vi "6 - Get transition sequence data from XY data.vi"() -> ()   [LabVIEW 2013]
uses:
  <vilib>/Utility/file.llb/Read From Spreadsheet File (DBL).vi
panel:
  out "Array":string[][](array[string])
  in  "video number":i32
  in  "startend data":path
  in  "player xy and frame data":path
  in  "player transition data":path
  in  "Number of transitions":i32=5
  out "subpatterns out":string[](array[string])
  out "Sub patterns 2":string[](array[string])
  out "Sub patterns":string[](array[string])
  out "top":string[][](array[string])
  out "bottom":string[][](array[string])
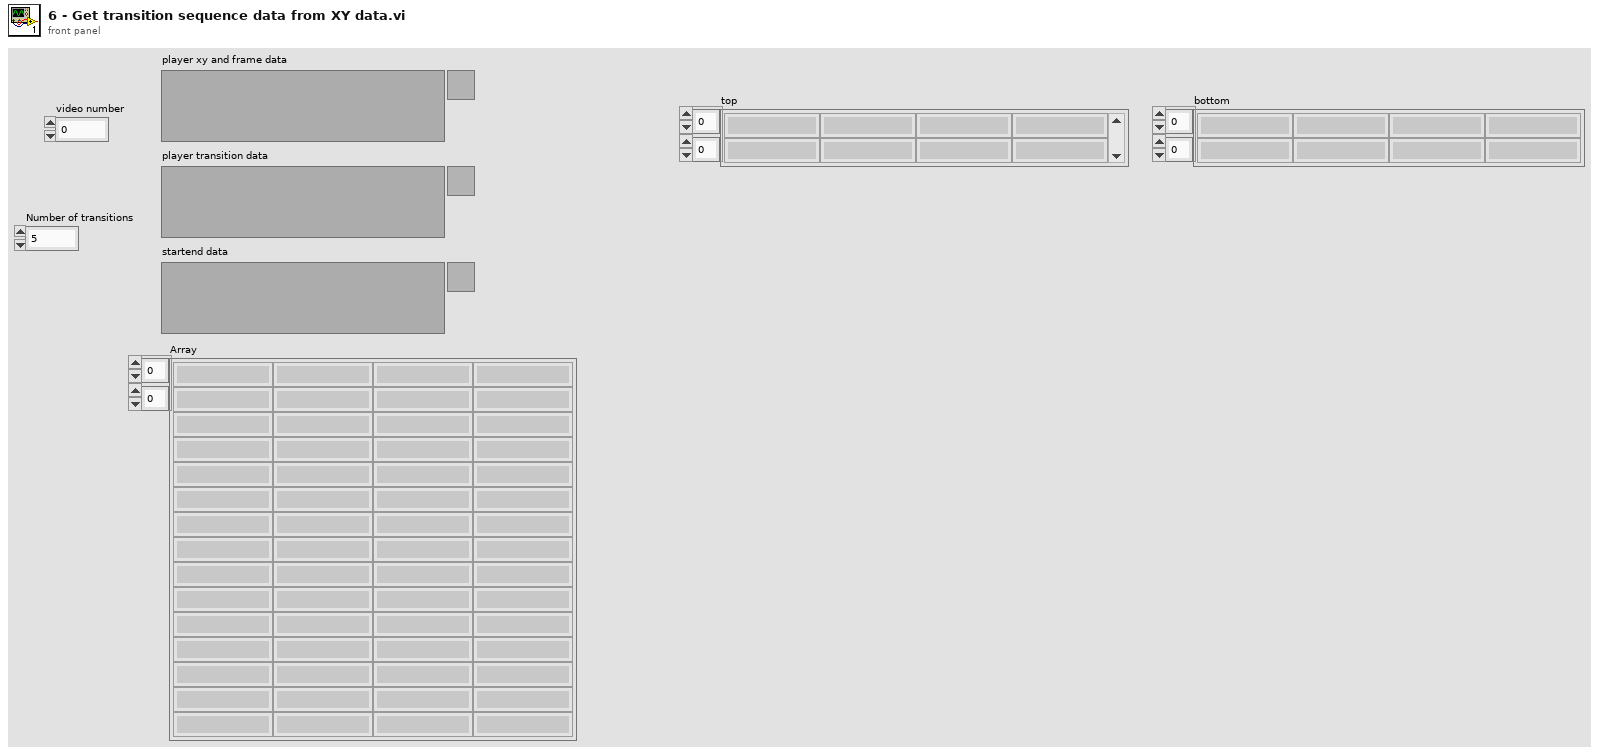
[diagram p1: front panel]
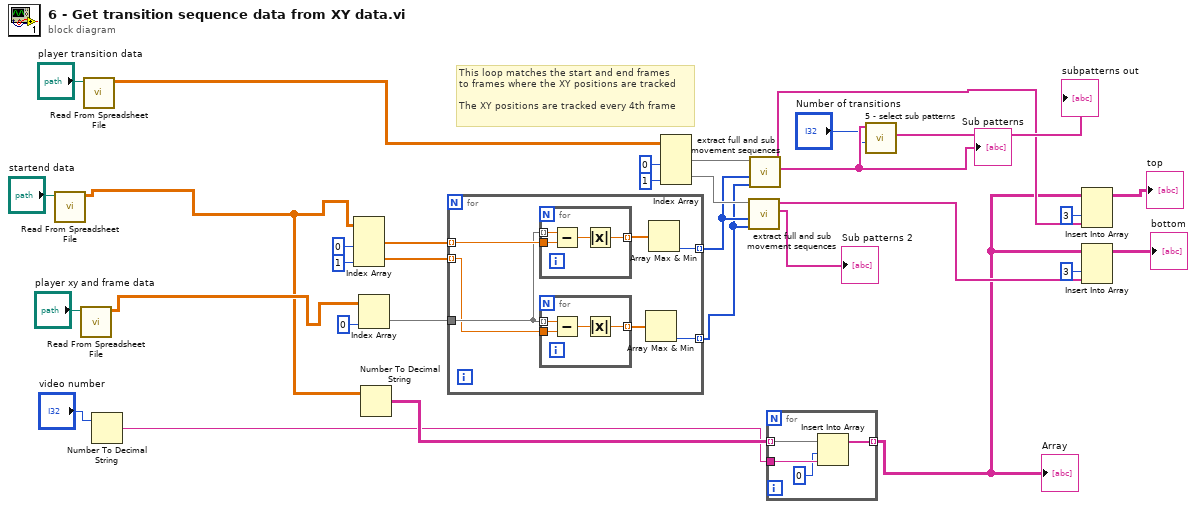
[diagram p0: block diagram]
diagram:
  # "This loop matches the start and end frames \nto frames where the XY positions are tracked\n\nThe XY positions are tracked every 4th frame"
  n1 = call-poly <vilib>:"Read From Spreadsheet File.vi"("file path (dialog if empty)"="startend data") -> ("all rows"=w11:dbl[][])  [unwired: 6 in, 4 out]
  n2 = call-poly <vilib>:"Read From Spreadsheet File.vi"("file path (dialog if empty)"="player xy and frame data") -> ("all rows"=w13:dbl[][])  [unwired: 6 in, 4 out]
  n3 = call-poly <vilib>:"Read From Spreadsheet File.vi"("file path (dialog if empty)"="player transition data") -> ("all rows"=w15:dbl[][])  [unwired: 6 in, 4 out]
  n4 = Number To Decimal String(number="video number") -> (decimal integer string=w8:string)  [unwired: 1 in]
  n5 = Index Array(array=w11, index (col) #1=0 ("disabled index (col)"), index (col) #2=1 ("index (col)")) -> (element #1=w30:dbl[], element #2=w29:dbl[])  [unwired: 2 in]
  n6 = Index Array(array=w13, index (col)=0 ("disabled index (col)")) -> (element=w27:dbl[])  [unwired: 1 in]
  n7 = Number To Decimal String(number=w11) -> (decimal integer string=w9:string[][])  [unwired: 1 in]
  n8 = for {
    tunnel: w30 -> [w39] mode=indexing
    tunnel: w29 -> [w34] mode=indexing
    tunnel: w27 -> [w35]
    tunnel: [w37] -> w22 mode=indexing
    tunnel: [w36] -> w21 mode=indexing
    n9 = for {
      tunnel: w39 -> [w46]
      tunnel: w35 -> [w47] mode=indexing
      tunnel: [w44] -> w38 mode=indexing
      n10 = Subtract(x=w47, y=w46) -> (x-y=w45:dbl)
      n11 = Absolute Value(x=w45) -> (abs(x)=w44:dbl)
    }
    n12 = for {
      tunnel: w34 -> [w42]
      tunnel: w35 -> [w43] mode=indexing
      tunnel: [w40] -> w33 mode=indexing
      n13 = Subtract(x=w43, y=w42) -> (x-y=w41:dbl)
      n14 = Absolute Value(x=w41) -> (abs(x)=w40:dbl)
    }
    n15 = Array Max & Min(array=w33) -> (min index (indices)=w36:i32)  [unwired: 3 out]
    n16 = Array Max & Min(array=w38) -> (min index (indices)=w37:i32)  [unwired: 3 out]
  }
  n17 = Index Array(array=w15, index (col) #1=0 ("disabled index (col)"), index (col) #2=1 ("index (col)")) -> (element #1=w24:dbl[], element #2=w23:dbl[])  [unwired: 2 in]
  n18 = call "extract full and sub movement sequences.vi"("end points in"=w21, "Start points in"=w22, "player movement data"=w23) -> ("Sub patterns"=→"Sub patterns 2":string[], "Full movement patterns"=w7:string[])  [unwired: 7 in]
  n19 = call "extract full and sub movement sequences.vi"("end points in"=w21, "Start points in"=w22, "player movement data"=w24) -> ("Sub patterns"=w19:string[], "Full movement patterns"=w3:string[])  [unwired: 7 in]
  "Sub patterns" <- w19
  n20 = for {
    tunnel: w9 -> [w51] mode=indexing
    tunnel: w8 -> [w50]
    tunnel: [w49] -> w2 mode=indexing
    n21 = Insert Into Array(array=w51, index=0, new element=w50) -> (w49:string[])
  }
  "Array" <- w2
  n22 = call "5 - select sub patterns.vi"("Number of transitions"="Number of transitions", "All Sub patterns"=w19) -> ("sub patterns out"=→"subpatterns out":string[])  [unwired: 9 in]
  n23 = Insert Into Array(array=w2, index (col)=3 ("disabled index (col)"), new element=w3) -> (→"top":string[][])  [unwired: 1 in]
  n24 = Insert Into Array(array=w2, index (col)=3 ("disabled index (col)"), new element=w7) -> (→"bottom":string[][])  [unwired: 1 in]
